vi "RSSI Peak Averaging.vi"(10 "Reject Ratio, % (75)":i32=75, 11 "Raw RSSI Data":u8[](array[numeric]) format="%02x") -> (3 "Averaged Peak RSSI":u8)   [LabVIEW 2020]
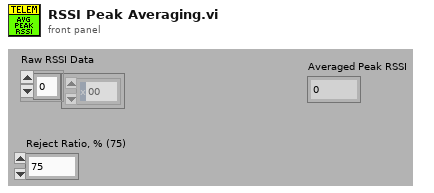
[diagram p1: front panel]
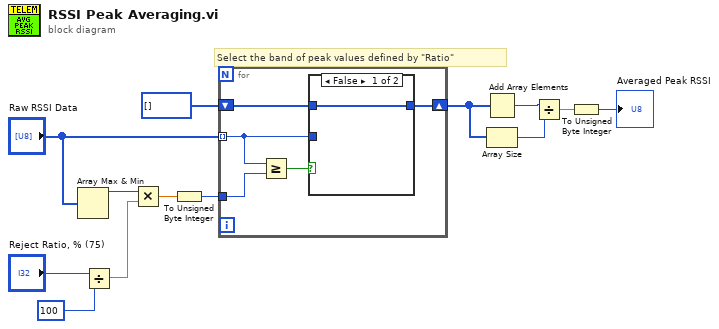
[diagram p0: block diagram]
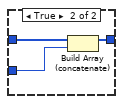
[diagram p2: hidden frame]
diagram:
  # "Select the band of peak values defined by \"Ratio\""
  n1 = Array Max & Min(array="Raw RSSI Data") -> (max value=w10:u8)  [unwired: 3 out]
  n2 = Divide(x="Reject Ratio, % (75)", y=100) -> (x/y=w9:dbl)
  n3 = Multiply(x=w10, y=w9) -> (x*y=w8:dbl)
  n4 = To Unsigned Byte Integer(number=w8) -> (unsigned 8bit integer=w7:u8)
  n5 = for {
    tunnel: "Raw RSSI Data" -> [w15] mode=indexing
    tunnel: w7 -> [w14]
    shift-right: [w17] -> w5
    shift-left: u8[] [] ("Raw RSSI Data") -> [w18]
    n6 = Greater Or Equal?(x=w15, y=w14) -> (x >= y?=w16:bool)
    n7 = case shown="False" w16 {
      tunnel: w15 -> [_ w20]
      tunnel: w18 -> [w19 w22]
      tunnel: [w19 w21] -> w17
      frame False {
      }
      frame True {
        n8 = Build Array (concatenate)(w22, w20) -> (w21:u8[])
      }
    }
  }
  n9 = Add Array Elements(numeric array=w5) -> (sum=w4:u8)
  n10 = Array Size(array=w5) -> (size(s)=w3:i32)
  n11 = Divide(x=w4, y=w3) -> (x/y=w2:dbl)
  n12 = To Unsigned Byte Integer(number=w2) -> (unsigned 8bit integer=→"Averaged Peak RSSI":u8)
